vi "Grava_summaryACQ.vi"(3 "sufix number":u32, 4 "ChipID list":u32[](array[numeric]) format="%x", 5 "ACQ full DATA file path":path caption="File path") -> (1 "quants events per chip":u32[](array[numeric]), 2 "suffixed file path":path)   [LabVIEW 2015, in "VIPM2.lvlib"]
doc: "Make and save ACQ summary.\nLlista events per ChipID."
uses:
  VIPM2.lvlib
panel:
  out "Barra Load events":i32(slide) scale=-1.0..400000.0
  # "Summarizing events per chip"
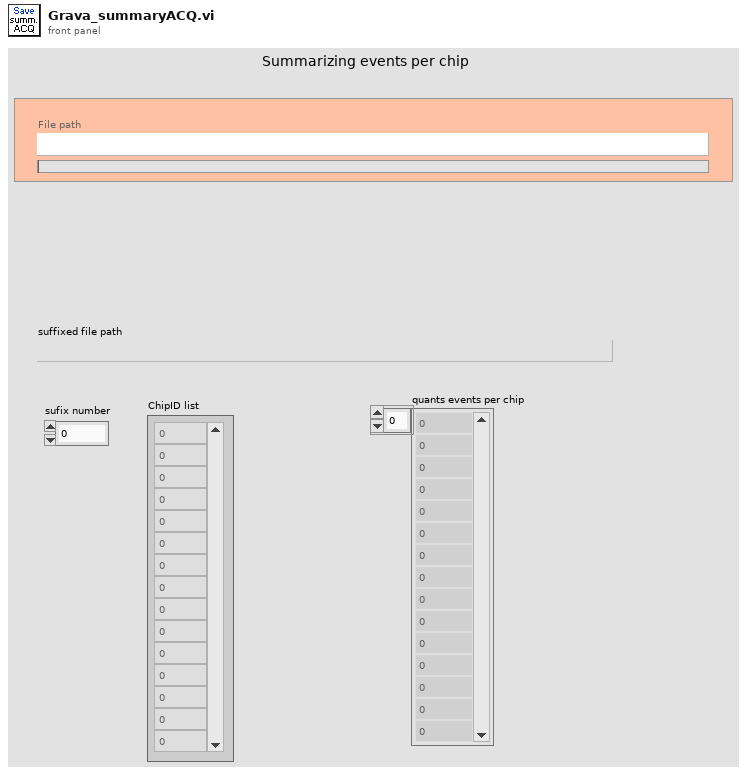
[diagram p1: front panel]
types:
  T1 = enum16{"big-endian, network order", "native, host order", "little-endian"}
  T2 = enum16{"open", "replace", "create", "open or create", "replace or create", "replace or create with confirmation"}
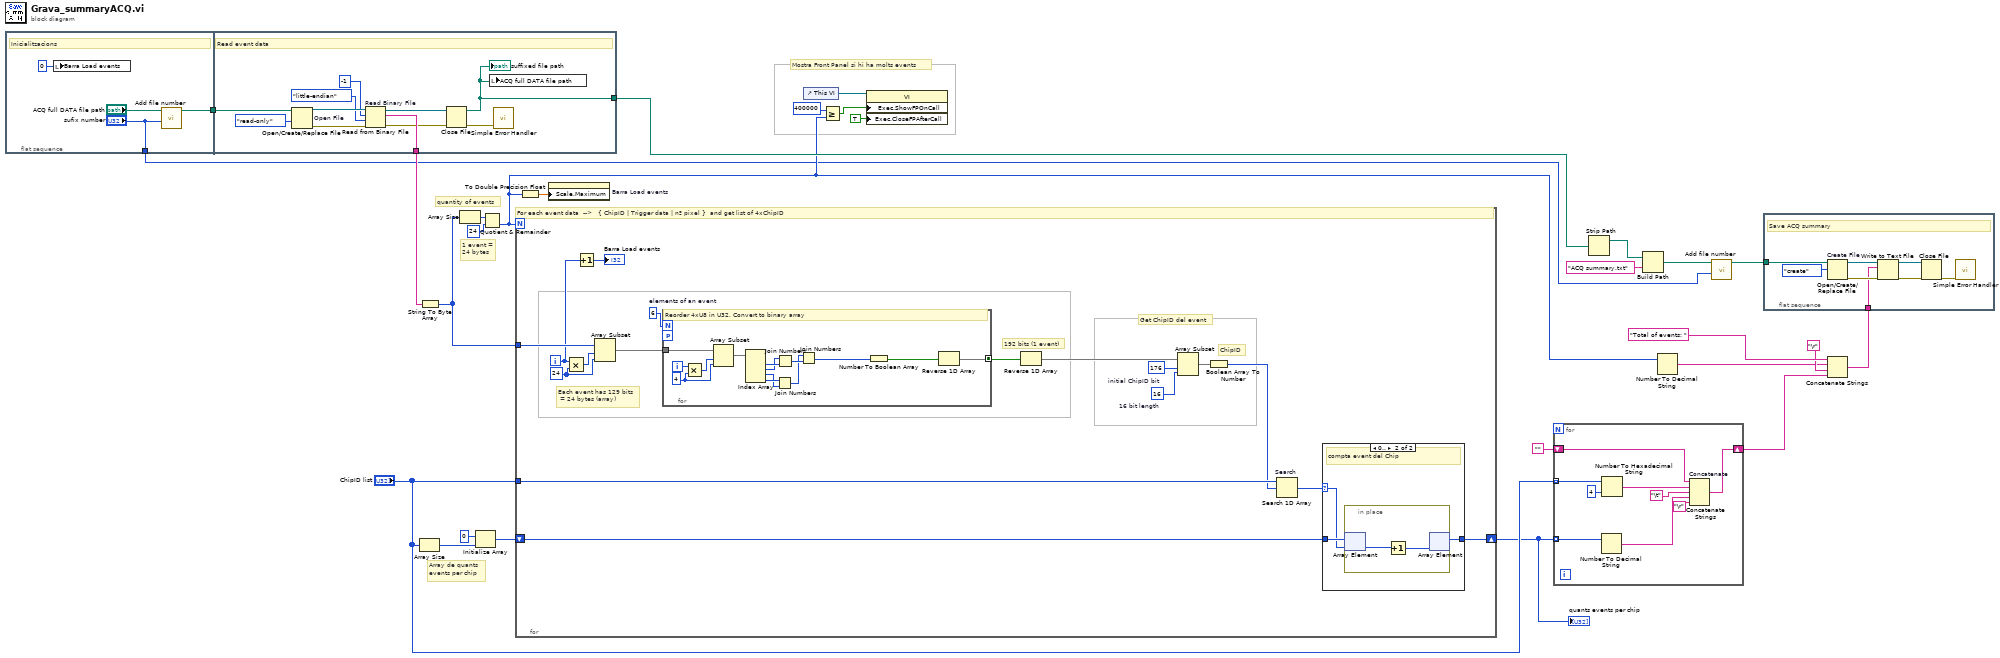
[diagram p0: block diagram]
diagram:
  # "Mostra Front Panel si hi ha molts events"
  # "Array de quants\nevents per chip"
  # "1 event =\n24 bytes"
  # "quantity of events"
  n1 = flat-sequence {
    tunnel: [w31] -> w23
    tunnel: ["sufix number"] -> w1
    tunnel: [w40] -> w25
    tunnel: w23 -> [w41]
    tunnel: [w33] -> w15
    frame #0 {
      # "Inicialitzacions"
      n2 = local write "Barra Load events"(0 ("Total number of events")) -> ()
      n3 = call "Add file number.vi"("sufix number"="sufix number", "file path"="ACQ full DATA file path") -> ("incremented file path"=w31:path)  [unwired: 9 in]
    }
    frame #1 {
      # "Read event data"
      n4 = Open/Create/Replace File "Open File"(file path (use dialog)=w41, access (0:read/write)=enum16{"read/write", "read-only", "write-only"}."read-only") -> (refnum out=w42:refnum<file>, error out=w43:errorcluster)  [unwired: 4 in, 1 out]
      n5 = Read from Binary File "Read Binary File"(8:w43, 9:T1."little-endian" ("byte order (0:big-endian, network order)"), 10:-1 ("count (1)"), 11:w42) -> (0:w37:errorcluster, 2:w40:string, 3:w36:refnum<file>)  [unwired: 2 in, 1 out]
      n6 = Close File(refnum=w36, error in=w37) -> (path=w33:path, error out=w34:errorcluster)
      "suffixed file path" <- w33
      n7 = local write "ACQ full DATA file path"(w33) -> ()
      n8 = call <vilib>:"Simple Error Handler.vi"("error in (no error)"=w34) -> ()  [unwired: 4 in, 5 out]
    }
  }
  n9 = Array Size(array="ChipID list") -> (size(s)=w22:i32)
  n10 = String To Byte Array(string=w25) -> (unsigned byte array=w26:u8[])
  n11 = Array Size(array=w26) -> (size(s)=w27:i32)
  n12 = Initialize Array "Initialize Array"(u32 0, w22) -> (w20:u32[])
  n13 = Quotient & Remainder(x=w27, y=24) -> (floor(x/y)=w6:i32)  [unwired: 1 out]
  n14 = for {
    N: w6 -> [_]
    tunnel: w26 -> [w56]
    tunnel: "ChipID list" -> [w48]
    shift-right: [w44] -> w16
    shift-left: w20 -> [w45]
    i -> [w52]
    w50 = 16  # 16 bit length
    w49 = 176  # initial ChipID bit
    w59 = 24 ("y")
    w60 = 6  # elements of an event
    # "Get ChipID del event"
    # "ChipID"
    # "192 bits (1 event)"
    # "Each event has 129 bits\n = 24 bytes (array)"
    # "For each event data  -->   { ChipID | Trigger data | nº pixel }  and get list of 4xChipID"
    n15 = Multiply(x=w52, y=w59) -> (x*y=w58:i32)
    n16 = Increment(x=w52) -> (x+1=→"Barra Load events":i32)
    n17 = Array Subset "Array Subset"(array=w56, index=w58, length=w59) -> (w57:u8[])
    n18 = for {
      N: w60 -> [_]
      tunnel: w57 -> [w79]
      workers-P: _ -> [_]
      tunnel: [w67] -> w55 mode=concatenating
      i -> [w80]
      w77 = 4 ("y")
      # "Reorder 4xU8 in U32. Convert to binary array"
      n19 = Multiply(x=w80, y=w77) -> (x*y=w78:i32)
      n20 = Array Subset "Array Subset"(array=w79, index=w78, length=w77) -> (w76:u8[])
      n21 = Index Array(array=w76) -> (element #1=w75:u8, element #2=w74:u8, element #3=w72:u8, element #4=w73:u8)  [unwired: 4 in]
      n22 = Join Numbers(hi=w73, lo=w72) -> ((hi.lo)=w70:u16)
      n23 = Join Numbers(hi=w74, lo=w75) -> ((hi.lo)=w71:u16)
      n24 = Join Numbers(hi=w70, lo=w71) -> ((hi.lo)=w68:u32)
      n25 = Number To Boolean Array(number=w68) -> (Boolean array=w69:bool[])
      n26 = Reverse 1D Array(array=w69) -> (reversed array=w67:bool[])
    }
    n27 = Reverse 1D Array(array=w55) -> (reversed array=w54:bool[])
    n28 = Array Subset "Array Subset"(array=w54, index=w49, length=w50) -> (w51:bool[])
    n29 = Boolean Array To Number(Boolean array=w51) -> (number=w47:u32)
    n30 = Search 1D Array "Search"(1D array=w48, element=w47) -> (index of element=w46:i32)  [unwired: 1 in]
    n31 = case shown="0.." w46 {
      selector: w46 -> [_ w63]
      tunnel: w45 -> [w61 w64]
      tunnel: [w61 w62] -> w44
      frame ..-1, Default {
        # "event d'un Chip no llistat"
      }
      frame 0.. {
        # "compta event del Chip"
        n32 = in-place "In Place Element Structure" {
          n33 = in-place-array #1(w64, w63) -> (w66:u32)
          n34 = Increment(x=w66) -> (x+1=w65:u32)
          n35 = in-place-array #1(w65) -> (w62:u32[])  [unwired: 1 out]
        }
      }
    }
  }
  "quants events per chip" <- w16
  n36 = To Double Precision Float(number=w6) -> (double precision float=w24:dbl)
  n37 = property on="Barra Load events" class="Slide (strict)"("Scale.Maximum"=w24) -> ()  [unwired: 2 in, 2 out]
  n38 = control-ref of="This VI"() -> (w8:refnum<vi>)
  n39 = Greater Or Equal?(x=400000, y=w6) -> (x >= y?=w7:bool)
  n40 = property class="VI"(reference=w8, "Exec.ShowFPOnCall"=w7, "Exec.CloseFPAfterCall"=TRUE ("Execution:Close After Call")) -> ()  [unwired: 1 in, 2 out]
  n41 = for {
    tunnel: "ChipID list" -> [w89] mode=indexing
    tunnel: w16 -> [w87] mode=indexing
    shift-right: [w81] -> w12
    shift-left: "" -> [w82]
    n42 = Number To Decimal String(number=w87) -> (decimal integer string=w84:string)  [unwired: 1 in]
    n43 = Number To Hexadecimal String(1:i16 4 ("width (-)"), 2:w89) -> (0:w86:string)
    n44 = Concatenate Strings "Concatenate"(w82, w86, "\t", w84, "\r") -> (w81:string)
  }
  n45 = Strip Path(path=w15) -> (stripped path=w14:path)  [unwired: 1 out]
  n46 = Build Path(base path=w14, name or relative path="ACQ summary.txt") -> (appended path=w3:path)
  n47 = Number To Decimal String(number=w6) -> (decimal integer string=w9:string)  [unwired: 1 in]
  n48 = call "Add file number.vi"("sufix number"=w1, "file path"=w3) -> ("incremented file path"=w2:path)  [unwired: 9 in]
  n49 = flat-sequence {
    tunnel: w2 -> [w97]
    tunnel: w18 -> [w90]
    frame #0 {
      # "Save ACQ summary"
      n50 = Open/Create/Replace File "Create File"(file path (use dialog)=w97, operation (0:open)=T2."create") -> (refnum out=w95:refnum<file>, error out=w94:errorcluster)  [unwired: 4 in, 1 out]
      n51 = Write to Text File(file (use dialog)=w95, text=w90, error in=w94) -> (refnum out=w93:refnum<file>, error out=w92:errorcluster)  [unwired: 1 in, 1 out]
      n52 = Close File(refnum=w93, error in=w92) -> (error out=w91:errorcluster)  [unwired: 1 out]
      n53 = call <vilib>:"Simple Error Handler.vi"("error in (no error)"=w91) -> ()  [unwired: 4 in, 5 out]
    }
  }
  n54 = Concatenate Strings "Concatenate Strings"("Total of events: " ("name or relative path"), w9, "\r", w12) -> (w18:string)
